vi "Get Playback Frame Data.vi"(8 "Error In":errorcluster, 10 "Frame number":u32, 11 "Frame Grabber Data":T1={"Camera Session"="", "Frame"=refnum, "AVI Refnum"=refnum, "Codecs"=[], "Frame number"=0, "Tracking File Refnum"=refnum, "Tick Count"=0, "Probe Object"=refnum, "Playback Probe Data"=[], "Rigid Body"={"Position"={"x (mm)"=0.0, "y (mm)"=0.0, "z (mm)"=0.0}, "Orientation"={"Pitch (rad)"=0.0, "Yaw (rad)"=0.0, "Roll (rad)"=0.0}, "Quaternion"={"qx"=0.0, "qy"=0.0, "qz"=0.0, "qw"=0.0}, "Tracked?"=FALSE}, "Total no frames playback"=0, "Video FPS"=0.0, "Camera connected?"=FALSE, "Scene"=refnum, "Cropped Frame"=refnum, "Tracker FPS"=0.0, "Crop ROI"=[], "Presentation Values"=[], "Elapsed time (ms)"=0, "Camera frames playback"=0, "Refnums"={"Live Refnum"=refnum, "Record Refnum"=refnum, "Recording Settings Refnum"=refnum, "Playback Refnum"=refnum, "Frame Slider Refnum"=refnum, "Pause Refnum"=refnum, "Home Refnum"=refnum, "Crop Refnum"=refnum, "Clear Crop Refnum"=refnum, "stop refnum"=refnum, "Playback Rate Refnum"=refnum, "Operator Settings Refnums"=refnum, "Presentation Refnum"=refnum, "Gestation Refnum"=refnum, "Crop Time Frame Slider Refnum"=refnum, "Cancel Save Refnum"=refnum, "Reverse Playback Refnum"=refnum, "Connection Settings Refnum"=refnum}, "Dimensions"={"Probe Dimensions"={"Probe Width"=0.0, "Probe Depth"=1.0, "Probe Height"=0.0}, "Room Dimensions"={"Room Width"=0.0, "Room Depth"=0.0, "Room Height"=0.0}}, "Playback Data As Strings"=[], "Cropped Tracking File Refnum"=refnum, "Cropped AVI Refnum"=refnum, "Header"=[], "Total euclidian distance"=0.0, "Annotation File Path"=path "", "Playback File Path"=path ""}) -> (0 "Error Out":errorcluster, 1 "Presentation":string, 2 "Time elapsed (s)":dbl, 3 "New Rigid Body Position":T5, 4 "Tracked?":bool)   [LabVIEW 2017]
uses:
  Controls/Rigid Body Info.ctl
  Controls/Position.ctl
  Controls/Orientation.ctl
  Controls/Frame Grabber Data.ctl
  <vilib>/userdefined/High Color/IMAQdx.ctl
  <vilib>/vision/Image Controls.llb/IMAQ Image.ctl
  <vilib>/vision/Avi.llb/IMAQ AVI2 Refnum.ctl
  Controls/Refnums.ctl
  Controls/Recording Settings.ctl
  Controls/Operator Settings.ctl
  Controls/Operator.ctl
  Controls/Connection Settings.ctl
  Controls/Tracker Type.ctl
  Controls/COM Port.ctl
  Controls/Dimensions.ctl
  Controls/Room Dimensions.ctl
  <vilib>/robotics/Kinematics/RotateX.vi
  <vilib>/robotics/Kinematics/RotateY.vi
  <vilib>/robotics/Kinematics/RotateZ.vi
  <vilib>/Analysis/baseanly.llb/A x B.vi
  <vilib>/Analysis/baseanly.llb/Real A x B.vi
  <vilib>/robotics/Kinematics/Rotation Matrix to Angle Vector.vi
  <vilib>/robotics/Kinematics/NI_Kinematics.lvlib
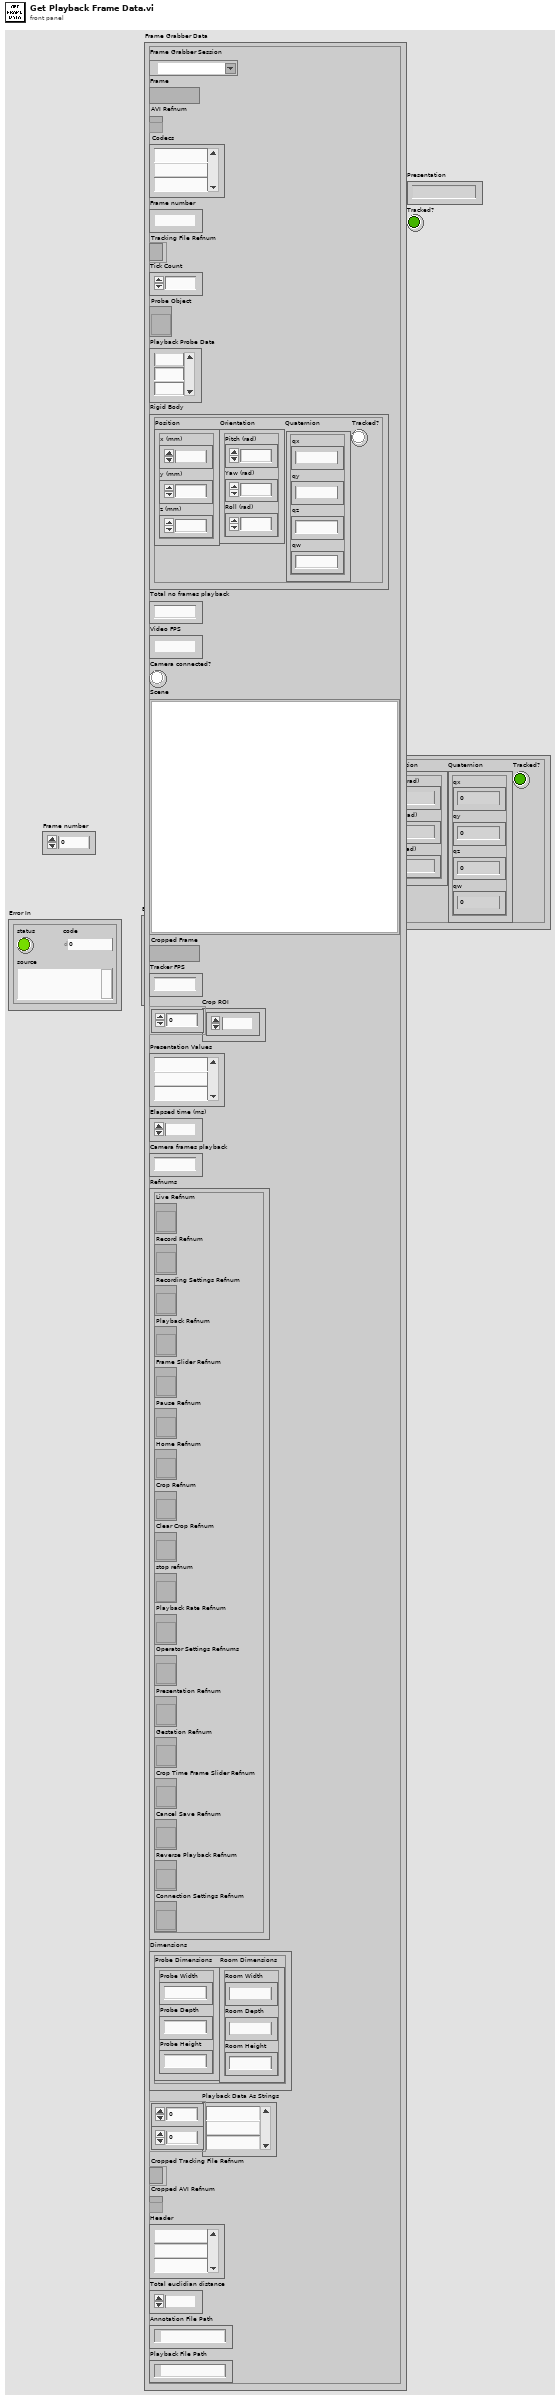
[diagram p1: front panel]
types:
  T1 = typedef "Frame Grabber Data.ctl" = cluster{"Camera Session":T2, "Frame":T3, "AVI Refnum":T4, "Codecs":string[], "Frame number":u32, "Tracking File Refnum":refnum<file>, "Tick Count":u32, "Probe Object":refnum<vi>, "Playback Probe Data":dbl[][], "Rigid Body":T5, "Total no frames playback":i32, "Video FPS":dbl, "Camera connected?":bool, "Scene":refnum<vi>, "Cropped Frame":T3, "Tracker FPS":dbl, "Crop ROI":i32[], "Presentation Values":string[], "Elapsed time (ms)":u32, "Camera frames playback":u32, "Refnums":T8, "Dimensions":T9, "Playback Data As Strings":string[][], "Cropped Tracking File Refnum":refnum<file>, "Cropped AVI Refnum":T4, "Header":string[], "Total euclidian distance":dbl, "Annotation File Path":path, "Playback File Path":path}
  T2 = typedef "IMAQdx.ctl" = refnum<k21>
  T3 = typedef "IMAQ Image.ctl" = refnum<image>
  T4 = typedef "IMAQ AVI2 Refnum.ctl" = refnum<k20>
  T5 = typedef "Rigid Body Info.ctl" = cluster{"Position":T6, "Orientation":T7, "Quaternion":cluster{"qx":sgl, "qy":sgl, "qz":sgl, "qw":sgl}, "Tracked?":bool}
  T6 = typedef "Position.ctl" = cluster{"x (mm)":sgl, "y (mm)":sgl, "z (mm)":sgl}
  T7 = typedef "Orientation.ctl" = cluster{"Pitch (rad)":sgl, "Yaw (rad)":sgl, "Roll (rad)":sgl}
  T8 = typedef "Refnums.ctl" = cluster{"Live Refnum":refnum<vi>, "Record Refnum":refnum<vi>, "Recording Settings Refnum":refnum<vi>, "Playback Refnum":refnum<vi>, "Frame Slider Refnum":refnum<vi>, "Pause Refnum":refnum<vi>, "Home Refnum":refnum<vi>, "Crop Refnum":refnum<vi>, "Clear Crop Refnum":refnum<vi>, "stop refnum":refnum<vi>, "Playback Rate Refnum":refnum<vi>, "Operator Settings Refnums":refnum<vi>, "Presentation Refnum":refnum<vi>, "Gestation Refnum":refnum<vi>, "Crop Time Frame Slider Refnum":refnum<vi>, "Cancel Save Refnum":refnum<vi>, "Reverse Playback Refnum":refnum<vi>, "Connection Settings Refnum":refnum<vi>}
  T9 = typedef "Dimensions.ctl" = cluster{"Probe Dimensions":cluster{"Probe Width":sgl, "Probe Depth":sgl, "Probe Height":sgl}, "Room Dimensions":T10}
  T10 = typedef "Room Dimensions.ctl" = cluster{"Room Width":dbl, "Room Depth":dbl, "Room Height":dbl}
  T11 = typedef "NI_Matrix.lvlib/RealMatrix.ctl" = dbl[][]
  T12 = typedef "NI_Kinematics.lvlib/Quaternion.ctl" = dbl[]
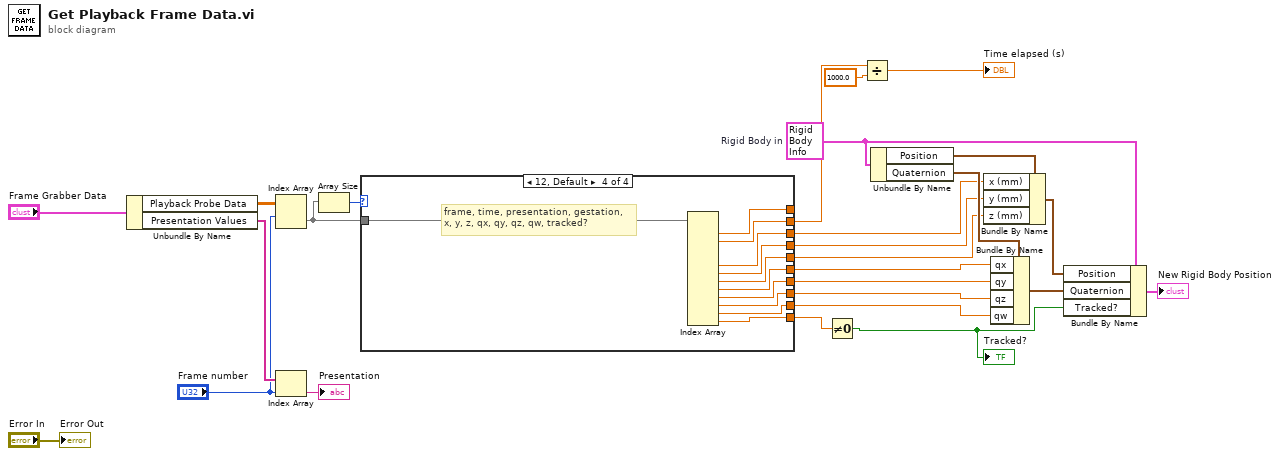
[diagram p0: block diagram]
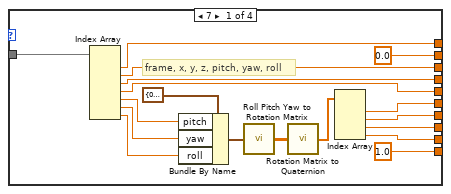
[diagram p2: hidden frame]
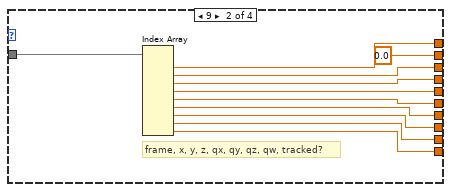
[diagram p3: hidden frame]
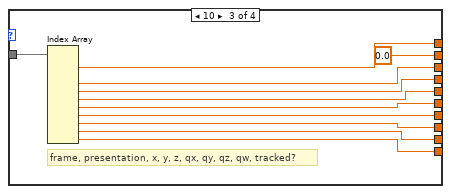
[diagram p4: hidden frame]
diagram:
  w18 = T5 {"Position"={"x (mm)"=0.0, "y (mm)"=0.0, "z (mm)"=0.0}, "Orientation"={"Pitch (rad)"=0.0, "Yaw (rad)"=0.0, "Roll (rad)"=0.0}, "Quaternion"={"qx"=0.0, "qy"=0.0, "qz"=0.0, "qw"=0.0}, "Tracked?"=FALSE}  # Rigid Body in
  n1 = Unbundle By Name("Frame Grabber Data") -> ("Playback Probe Data"=w5:dbl[][], "Presentation Values"=w4:string[])
  n2 = Index Array(array=w5, index (row)="Frame number") -> (element=w23:dbl[])  [unwired: 1 in]
  n3 = Index Array(array=w4, index="Frame number") -> (element=→"Presentation":string)
  n4 = Array Size(array=w23) -> (size(s)=w24:i32)
  n5 = case shown="12, Default" w24 {
    tunnel: w23 -> [w44 w55 w66 w77]
    tunnel: [w41 w54 w63 w74] -> w7
    tunnel: [w40 w53 w62 w73] -> w8
    tunnel: [w39 w52 w61 w72] -> w9
    tunnel: [w30 w51 w60 w71] -> w10
    tunnel: [w29 w50 w59 w70] -> w11
    tunnel: [w28 w49 w58 w69] -> w12
    tunnel: [w27 w48 w57 w68] -> w19
    tunnel: [1.0 ("Numeric") w47 w56 w67] -> w20
    tunnel: [w43 w45 w65 w76] -> _
    tunnel: [0.0 ("Numeric") 0.0 ("Numeric") 0.0 ("Numeric") w75] -> w22
    frame 7 {
      # "frame, x, y, z, pitch, yaw, roll"
      n6 = Index Array(array=w44) -> (element #1=w43:dbl, element #2=w41:dbl, element #3=w40:dbl, element #4=w39:dbl, element #5=w33:dbl, element #6=w31:dbl, element #7=w32:dbl)  [unwired: 7 in]
      n7 = Bundle By Name(cluster=cluster{"roll":dbl, "pitch":dbl, "yaw":dbl} {"roll"=0.0, "pitch"=0.0, "yaw"=0.0} ("angles"), "pitch"=w33, "yaw"=w31, "roll"=w32) -> (w38:cluster{"roll":dbl, "pitch":dbl, "yaw":dbl})
      n8 = call <vilib>:"Roll Pitch Yaw to Rotation Matrix.vi"("angles"=w38) -> ("rotation matrix"=w36:T11)
      n9 = call <vilib>:"Rotation Matrix to Quaternion.vi"("rotation matrix"=w36) -> ("quaternion"=w35:T12)
      n10 = Index Array(array=w35) -> (element #1=w30:dbl, element #2=w29:dbl, element #3=w28:dbl, element #4=w27:dbl)  [unwired: 4 in]
    }
    frame 9 {
      # "frame, x, y, z, qx, qy, qz, qw, tracked?"
      n11 = Index Array(array=w55) -> (element #1=w45:dbl, element #2=w54:dbl, element #3=w53:dbl, element #4=w52:dbl, element #5=w51:dbl, element #6=w50:dbl, element #7=w49:dbl, element #8=w48:dbl, element #9=w47:dbl)  [unwired: 9 in]
    }
    frame 10 {
      # "frame, presentation, x, y, z, qx, qy, qz, qw, tracked?"
      n12 = Index Array(array=w66) -> (element #1=w65:dbl, element #3=w63:dbl, element #4=w62:dbl, element #5=w61:dbl, element #6=w60:dbl, element #7=w59:dbl, element #8=w58:dbl, element #9=w57:dbl, element #10=w56:dbl)  [unwired: 10 in, 1 out]
    }
    frame 12, Default {
      # "frame, time, presentation, gestation,\nx, y, z, qx, qy, qz, qw, tracked?"
      n13 = Index Array(array=w77) -> (element #1=w76:dbl, element #2=w75:dbl, element #5=w74:dbl, element #6=w73:dbl, element #7=w72:dbl, element #8=w71:dbl, element #9=w70:dbl, element #10=w69:dbl, element #11=w68:dbl, element #12=w67:dbl)  [unwired: 12 in, 2 out]
    }
  }
  n14 = Not Equal To 0?(x=w20) -> (x != 0?=w21:bool)
  "Tracked?" <- w21
  n15 = Divide(x=w22, y=1000.0) -> (x/y=→"Time elapsed (s)":dbl)
  n16 = Unbundle By Name(w18) -> ("Position"=w14:T6, "Quaternion"=w15:cluster{"qx":sgl, "qy":sgl, "qz":sgl, "qw":sgl})
  n17 = Bundle By Name(cluster=w14, "x (mm)"=w7, "y (mm)"=w8, "z (mm)"=w9) -> (w13:T6)
  n18 = Bundle By Name(cluster=w15, "qx"=w10, "qy"=w11, "qz"=w12, "qw"=w19) -> (w16:cluster{"qx":sgl, "qy":sgl, "qz":sgl, "qw":sgl})
  n19 = Bundle By Name(cluster=w18, "Position"=w13, "Quaternion"=w16, "Tracked?"=w21) -> (→"New Rigid Body Position":T5)
  "Error Out" <- "Error In"
